vi "Convert To Enum Array.vi"(1 "Numeric Input":u16[](array[numeric])) -> (0 "Enum Output":T1[](array[typedef]))   [LabVIEW 2014]
uses:
  Shared/Auton Functions.ctl
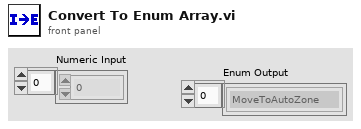
[diagram p1: front panel]
types:
  T1 = typedef "Auton Functions.ctl" = enum16{"MoveToAutoZone", "MoveToTote", "Pickup", "GrabRightCan", "GrabLeftCan", "SetThirdTote", "SetSecondTote", "SetFirstTote"}
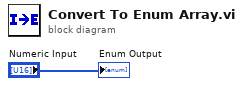
[diagram p0: block diagram]
diagram:
  "Enum Output" <- "Numeric Input"
